vi "TSM SSC Digital Init State.vi"(0 "Digital TSM In":T1, 5 "state":T3 items=["0"=0, "1"=1, "X"=5], 11 "error in":errorcluster) -> (4 "Digital TSM Out":T1, 15 "error out":errorcluster)   [LabVIEW 2019]
uses:
  <instrlib>/niDigital/niDigital.llb/niDigital Write Static Pin State.ctl
  TSM SSC Digital.ctl
  <vilib>/NI_TestStand_SemiconductorModule/NI_TestStand_Semiconductor_Module.lvlibp/PinMap/Digital Pattern/PinQueryContext/DigitalPatternPinQueryContext.lvclass
  SSC Digital/SSC Digital.ctl
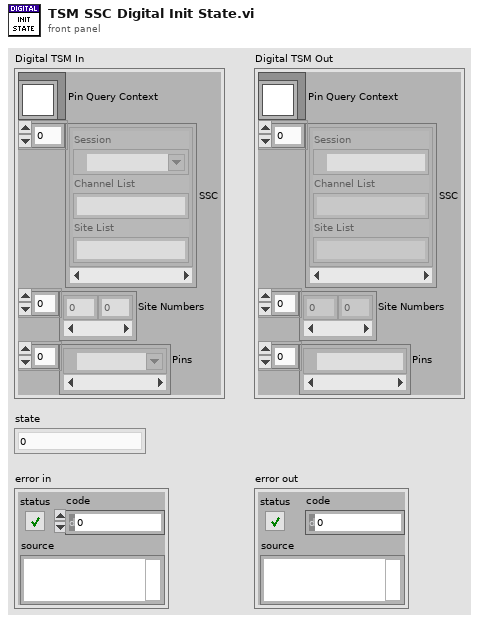
[diagram p1: front panel]
types:
  T1 = typedef "TSM SSC Digital.ctl" = cluster{"Pin Query Context":refnum<class "DigitalPatternPinQueryContext.lvclass">, "SSC":T2[], "Site Numbers":i32[], "Pins":tag[]}
  T2 = typedef "SSC Digital.ctl" = cluster{"Session":refnum<k15>, "Channel List":string, "Site List":string}
  T3 = typedef "niDigital Write Static Pin State.ctl" = u8
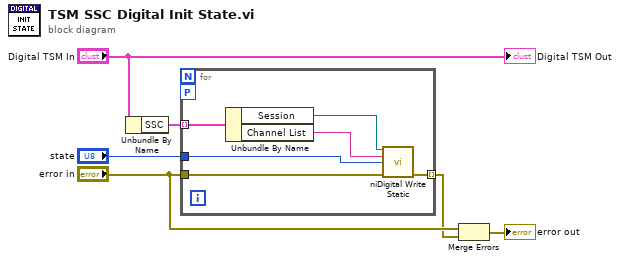
[diagram p0: block diagram]
diagram:
  n1 = Unbundle By Name("Digital TSM In") -> ("SSC"=w2:T2[])
  n2 = for {
    tunnel: "error in" -> [w12]
    tunnel: [w11] -> w4 mode=indexing
    workers-P: _ -> [_]
    tunnel: "state" -> [w10]
    tunnel: w2 -> [w9] mode=indexing
    n3 = Unbundle By Name(w9) -> ("Session"=w7:refnum<k15>, "Channel List"=w8:string)
    n4 = call <instrlib>:"niDigital Write Static.vi"("instrument handle"=w7, "channel list"=w8, "state"=w10, "error in"=w12) -> ("error out"=w11:errorcluster)  [unwired: 10 in, 1 out]
  }
  n5 = Merge Errors("error in", w4) -> (→"error out":errorcluster)
  "Digital TSM Out" <- "Digital TSM In"
